vi "Practica 13 - subCorriente.vi"(1 "I-Total":dbl, 2 "Ra":dbl, 3 "Rb":dbl) -> (0 "Ix":dbl)   [LabVIEW 2023]
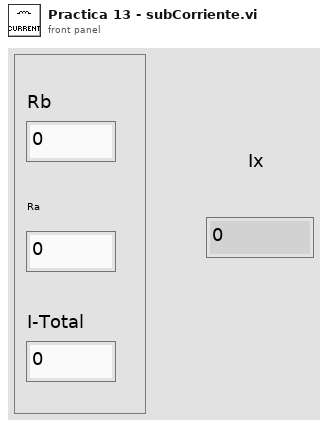
[diagram p1: front panel]
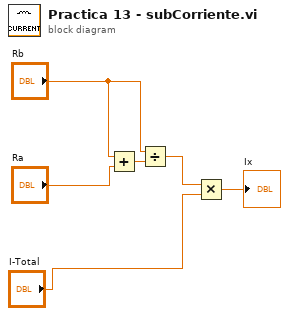
[diagram p0: block diagram]
diagram:
  n1 = Add(x="Rb", y="Ra") -> (x+y=w6:dbl)
  n2 = Divide(x="Rb", y=w6) -> (x/y=w2:dbl)
  n3 = Multiply(x=w2, y="I-Total") -> (x*y=→"Ix":dbl)
